vi "TDMS File Initialization (Read).vi"(8 "error in (no error)":errorcluster, 10 "Image In":T3, 11 "File Path":path) -> (0 "error out":errorcluster, 1 "Number of Images in TDMS File":u32, 2 "Read Settings":T1 {"Image Type" items=["Grayscale (U8)", "Grayscale (I16)", "Grayscale (SGL)", "Complex (CSG)", "RGB (U32)", "HSL (U32)", "RGB (U64)", "Grayscale (U16)"]}, 3 "TDMS Refnum Out":refnum<k34>)   [LabVIEW 2020]
uses:
  <vilib>/vision/Image Controls.llb/IMAQ Image.ctl
  TDMS Read Data.ctl
  TDMS Global.vi
panel:
  # "Overview:  Use this helper VI to initialize the settings for reading TDMS files that were written using the TDMS File Initialization (Write) VI.\n\nFile Path: Path to Open\nImage In: The image that will be updated when reading TDMS files. Make sure the data type of this image matches the data type of the images saved to the TDMS file.\n\nTDMS Refnum Out: The configured TDMS reference that can be used to TDMS files.\nRead Settings: Cluster should be passed to the TDMS Read File helper VI.\n   Image Type: Image type of image to be read\n   Width: The width of the image\n   Height: The height of the image\n   Pixels per Image: the number of pixels for each image, which can include border pixels and pixels used for padding.\n   Total Width: The width of the saved image, which includes border and padding.\n   Left Offset: The offset from the left side of the image to the first valid pixel of each row.\nNumber of Images in TDMS File: Number of images in TDMS File."
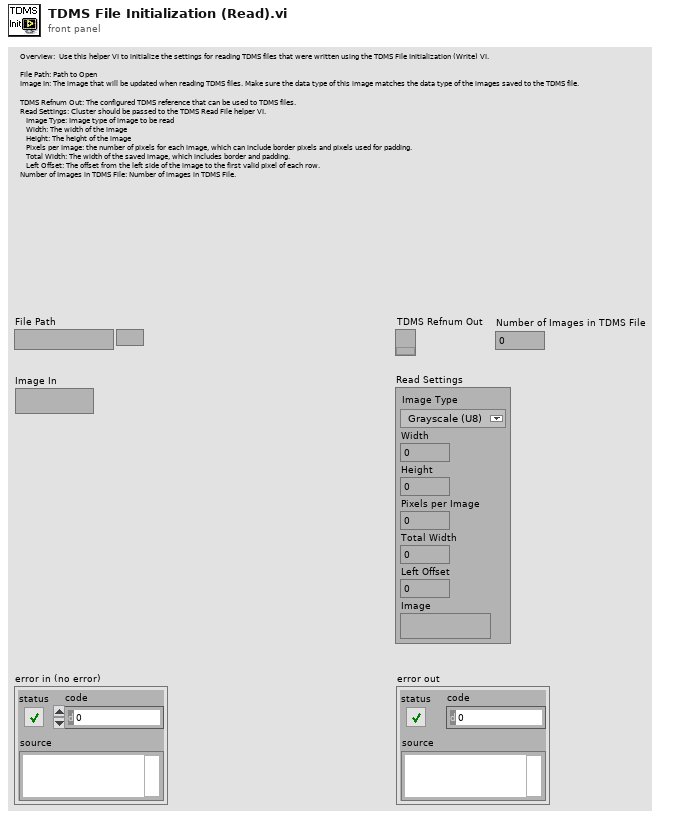
[diagram p1: front panel]
types:
  T1 = typedef "TDMS Read Data.ctl" = cluster{"Image Type":T2, "Width":u32, "Height":u32, "Pixels per Image":u32, "Total Width":u32, "Left Offset":u32, "Image":T3}
  T2 = typedef "Image Type" = u32
  T3 = typedef "IMAQ Image.ctl" = refnum<image>
  T4 = enum16{"open", "open or create", "create or replace", "create", "open (read-only)"}
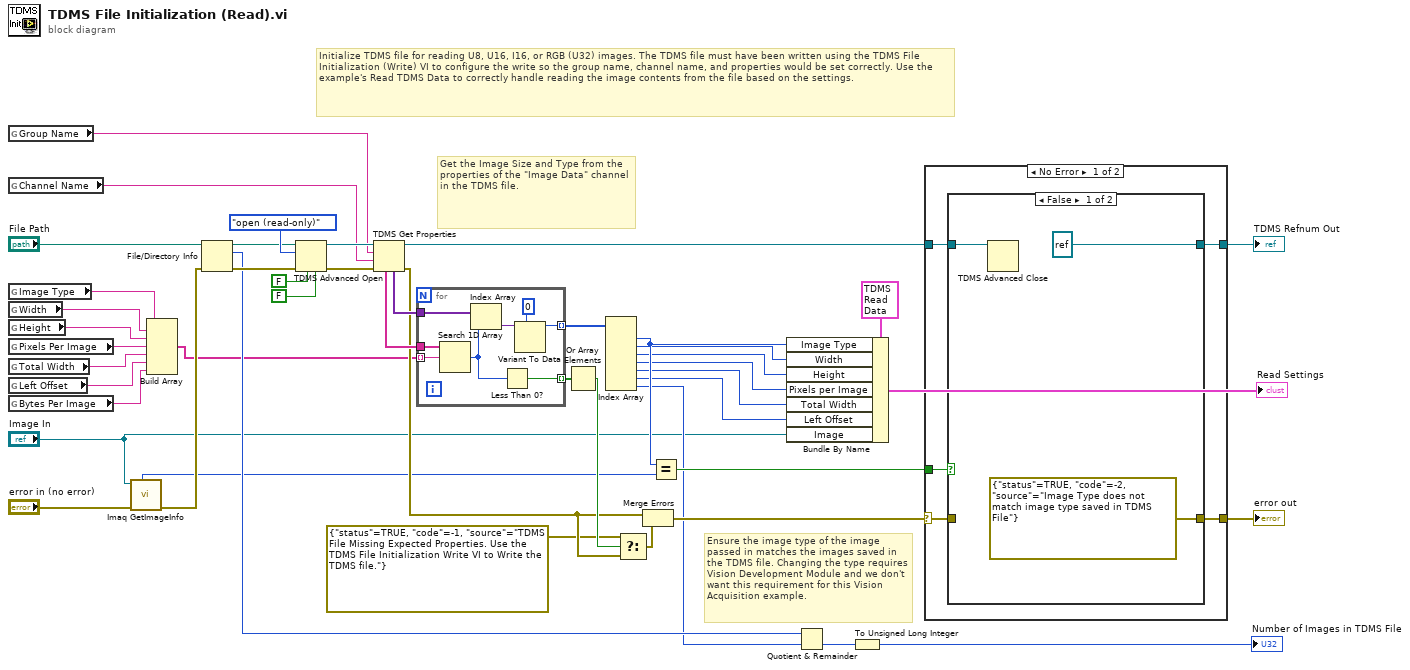
[diagram p0: block diagram]
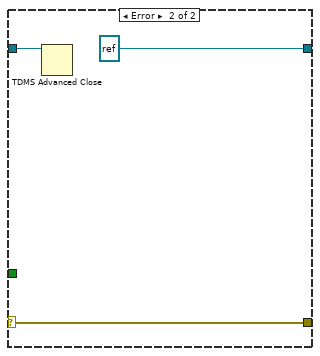
[diagram p3: hidden frame]
diagram:
  # "Initialize TDMS file for reading U8, U16, I16, or RGB (U32) images. The TDMS file must have been written using the TDMS File Initialization (Write) VI to configure the write so the group name, channel name, and properties would be set correctly. Use the example's Read TDMS Data to correctly handle reading the image contents from the file based on the settings."
  # "Get the Image Size and Type from the properties of the \"Image Data\" channel in the TDMS file."
  # "Ensure the image type of the image passed in matches the images saved in the TDMS file. Changing the type requires Vision Development Module and we don't want this requirement for this Vision Acquisition example."
  n1 = global read "TDMS Global.vi" "Group Name"() -> (w10:string)
  n2 = global read "TDMS Global.vi" "Channel Name"() -> (w9:string)
  n3 = global read "TDMS Global.vi" "Image Type"() -> (w5:string)
  n4 = global read "TDMS Global.vi" "Width"() -> (w6:string)
  n5 = global read "TDMS Global.vi" "Height"() -> (w7:string)
  n6 = global read "TDMS Global.vi" "Pixels Per Image"() -> (w8:string)
  n7 = global read "TDMS Global.vi" "Total Width"() -> (w4:string)
  n8 = global read "TDMS Global.vi" "Left Offset"() -> (w3:string)
  n9 = global read "TDMS Global.vi" "Bytes Per Image"() -> (w2:string)
  n10 = call "Imaq GetImageInfo"("error in (no error)"="error in (no error)", "Image"="Image In") -> ("error out"=w26:errorcluster, "Image Type"=w15:T2)  [unwired: 2 in, 6 out]
  n11 = Build Array(w5, w6, w7, w8, w4, w3, w2) -> (w1:string[])
  n12 = File/Directory Info(path="File Path", error in=w26) -> (path out=w27:path, size=w22:i64, error out=w25:errorcluster)  [unwired: 4 out]
  n13 = TDMS Advanced Open(4:FALSE ("disable buffering? (T)"), 6:FALSE ("disable buffering? (T)"), 8:w25, 10:T4."open (read-only)" ("operation (0:open)"), 11:w27) -> (0:w40:errorcluster, 3:w41:refnum<k34>)  [unwired: 1 out]
  n14 = TDMS Get Properties(8:w40, 9:w9, 10:w10, 11:w41) -> (0:w34:errorcluster, 3:w29:refnum<k34>, 4:w38:variant[], 6:w39:string[])  [unwired: 2 in, 2 out]
  n15 = for {
    tunnel: w1 -> [w54] mode=indexing
    tunnel: w39 -> [w55]
    tunnel: w38 -> [w53]
    tunnel: [w50] -> w37 mode=indexing
    tunnel: [w48] -> w36 mode=indexing
    n16 = Search 1D Array(1D array=w55, element=w54) -> (index of element=w49:i32)  [unwired: 1 in]
    n17 = Index Array(array=w53, index=w49) -> (element=w51:variant)
    n18 = Less Than 0?(x=w49) -> (x < 0?=w48:bool)
    n19 = Variant To Data(type=u32 0, Variant=w51) -> (data=w50:u32)  [unwired: 1 in, 1 out]
  }
  n20 = Or Array Elements(Boolean array=w36) -> (logical OR=w35:bool)
  n21 = Index Array(array=w37) -> (element #1=w20:u32, element #2=w19:u32, element #3=w18:u32, element #4=w17:u32, element #5=w16:u32, element #6=w13:u32, element #7=w14:u32)  [unwired: 7 in]
  n22 = Select(t=errorcluster {"status"=TRUE, "code"=-1, "source"="TDMS File Missing Expected Properties. Use the TDMS File Initialization Write VI to Write the TDMS file."}, s=w35, f=w34) -> (s? t:f=w32:errorcluster)
  n23 = Merge Errors(w34, w32) -> (w30:errorcluster)
  n24 = Equal?(x=w20, y=w15) -> (x = y?=w31:bool)
  n25 = Bundle By Name(cluster=T1 {"Image Type"=0, "Width"=640, "Height"=480, "Pixels per Image"=337920, "Total Width"=640, "Left Offset"=640, "Image"="test"} ("Read Settings"), "Image Type"=w20, "Width"=w19, "Height"=w18, "Pixels per Image"=w17, "Total Width"=w16, "Left Offset"=w13, "Image"="Image In") -> (→"Read Settings":T1)
  n26 = Quotient & Remainder(x=w22, y=w14) -> (floor(x/y)=w23:i64)  [unwired: 1 out]
  n27 = To Unsigned Long Integer(number=w23) -> (unsigned 32bit integer=→"Number of Images in TDMS File":u32)
  n28 = case shown="No Error" w30 {
    selector: w30 -> [w56 w68]
    tunnel: w29 -> [w60 w67]
    tunnel: [w59 refnum<k34> refnum ("tdms file out")] -> w47
    tunnel: [w58 w68] -> w46
    tunnel: w31 -> [w57 _]
    frame No Error {
      n29 = case shown="False" w57 {
        tunnel: w60 -> [w63 w65]
        tunnel: [refnum<k34> refnum ("tdms file out") w65] -> w59
        tunnel: [errorcluster {"status"=TRUE, "code"=-2, "source"="Image Type does not match image type saved in TDMS File"} ("error out") w64] -> w58
        tunnel: w56 -> [_ w64]
        frame False {
          n30 = TDMS Advanced Close(11:w63) -> ()  [unwired: 3 in, 2 out]
        }
        frame True {
        }
      }
    }
    frame Error {
      n31 = TDMS Advanced Close(11:w67) -> ()  [unwired: 3 in, 2 out]
    }
  }
  "TDMS Refnum Out" <- w47
  "error out" <- w46
